vi "Coord window-Parameter overwrite interlock.vi"(9 "Parameter name":string, 10 "Parameter's new value":i32, 11 "Parameter's old value":i32) -> (3 "Cancelled":bool)   [LabVIEW 2013]
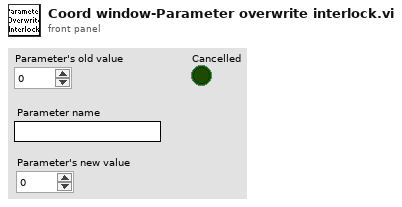
[diagram p1: front panel]
types:
  T1 = cluster{"Caption-Right button":string, "Caption-Left button":string, "Message to display":string, "Delay before close":u32, "Window Colour":u32, "Cancel button disabled?":enum8{"Enabled", "Disabled", "Disabled and Grayed Out"}}
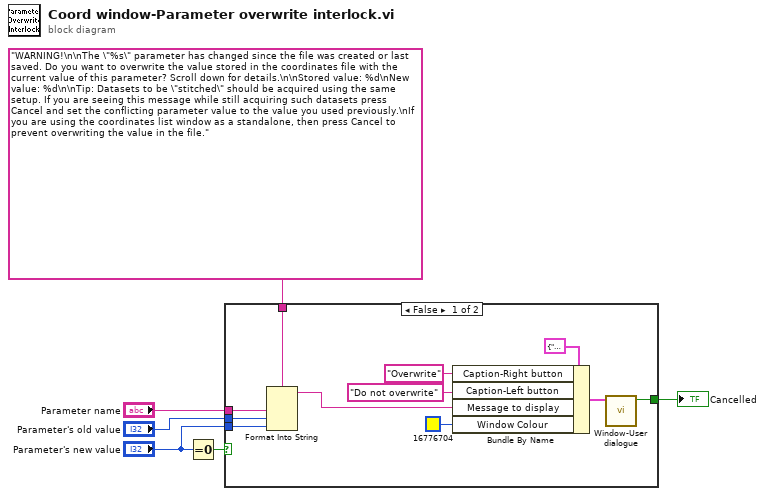
[diagram p0: block diagram]
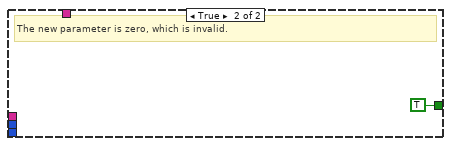
[diagram p2: hidden frame]
diagram:
  n1 = Equal To 0?(x="Parameter's new value") -> (x = 0?=w1:bool)
  n2 = case shown="False" w1 {
    tunnel: [w17 TRUE ("Left Button (Cancel)")] -> w6
    tunnel: "Parameter's old value" -> [w12 _]
    tunnel: "Parameter name" -> [w11 _]
    tunnel: "WARNING!\n\nThe \"%s\" parameter has changed since the file was created or last saved. Do you want to overwrite the value stored in the coordinates file with the current value of this parameter? Scroll down for details.\n\nStored value: %d\nNew value: %d\n\nTip: Datasets to be \"stitched\" should be acquired using the same setup. If you are seeing this message while still acquiring such datasets press Cancel and set the conflicting parameter value to the value you used previously.\nIf you are using the coordinates list window as a standalone, then press Cancel to prevent overwriting the value in the file." ("format string") -> [w10 _]
    tunnel: "Parameter's new value" -> [w7 _]
    frame False {
      n3 = Format Into String(format string=w10, w11, w12, w7) -> (resulting string=w8:string)  [unwired: 2 in, 1 out]
      n4 = Bundle By Name(cluster=T1 {"Caption-Right button"="", "Caption-Left button"="", "Message to display"="", "Delay before close"=0, "Window Colour"=16448250, "Cancel button disabled?"=enum."Enabled"} ("Input cluster"), "Caption-Right button"="Overwrite", "Caption-Left button"="Do not overwrite", "Message to display"=w8, "Window Colour"=u32 16776704) -> (w13:T1)
      n5 = call "Window-User dialogue.vi"("Input cluster"=w13) -> ("Left Button (Cancel)"=w17:bool)  [unwired: 10 in]
    }
    frame True {
      # "The new parameter is zero, which is invalid."
    }
  }
  "Cancelled" <- w6
